vi "Read plugin VI Refs.vi"(8 "error in (no error)":errorcluster, 11 "subpanel (abstract) in":refnum<class "subpanel (abstract).lvclass">) -> (0 "error out":errorcluster, 2 "plugin VI Refs":refnum<vi>[](array[refnum]), 3 "subpanel (abstract) out":refnum<class "subpanel (abstract).lvclass">)   [LabVIEW 2023, in "GUI.lvlib" / "subpanel (abstract).lvclass"]
uses:
  subpanel (abstract).lvclass
  subpanel (abstract).lvclass/subpanel (abstract).ctl
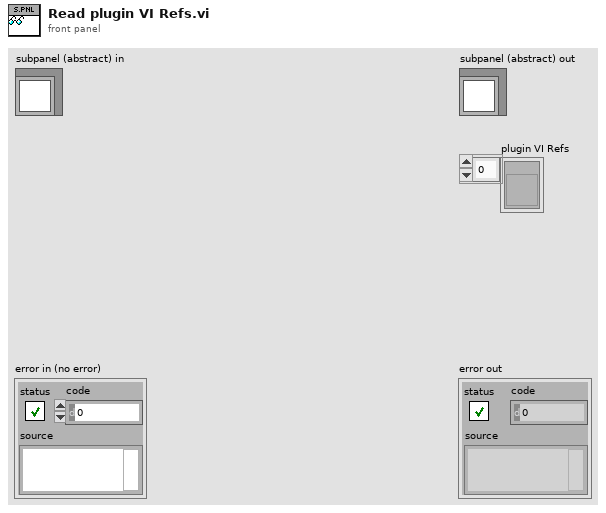
[diagram p1: front panel]
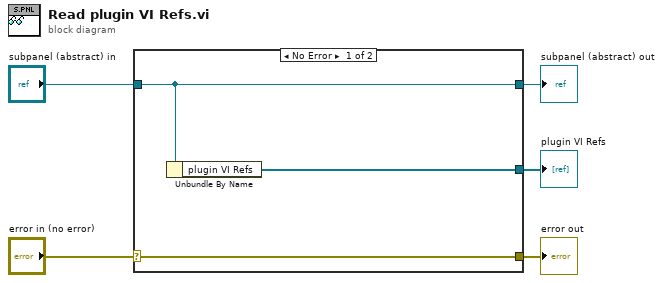
[diagram p0: block diagram]
diagram:
  n1 = case shown="No Error" "error in (no error)" {
    selector: "error in (no error)" -> [w8 w9]
    tunnel: [w8 w9] -> w4
    tunnel: [w7 w10] -> w2
    tunnel: "subpanel (abstract) in" -> [w7 w10]
    tunnel: [w6 _] -> w1
    frame No Error {
      n2 = Unbundle By Name(w7) -> ("plugin VI Refs"=w6:refnum<vi>[])
    }
    frame Error {
    }
  }
  "error out" <- w4
  "subpanel (abstract) out" <- w2
  "plugin VI Refs" <- w1
